vi "EloMec Tester.vi"() -> ()   [LabVIEW 2023]
uses:
  Communication_class/Paths/Convert AI Robot to Robot Command Folder/grSim/grSim Robot Command.ctl
  Communication_class/feedbackData.ctl
  <vilib>/Instr/_visa.llb/VISA Configure Serial Port (Instr).vi
  Communication_class/Communication.lvclass
panel:
  out "Waveform Chart 3":u32(graph)
  out "Waveform Chart 2":u32(graph)
  in  "Modo":T1(ring)
  out "Battery":sgl(graph)
  in  "Feedback ID":u32
  out "Space":bool
  out "kickCharged":bool
  out "hasBall":bool
  out "E":bool
  out "Q":bool
  in  "Keyboard":bool=TRUE
  out "A":bool
  out "D":bool
  out "S":bool
  out "W":bool
  in  "Zero":bool
  out "Waveform Chart":T2(graph)
  out "FeedbackData":T3 {"status" format="%08x"}
  in  "FIRASim?":bool
  in  "IDs":u32[](array[numeric])
  out "Output Array":T4[](array[typedef])=[{"id"=0, "kickspeedx"=0.0, "kickspeedz"=0.0, "veltangent"=0.0, "velnormal"=0.0, "velangular"=0.0, "spinner"=FALSE, "wheelspeed"=FALSE, "wheel1"=0.0, "wheel2"=0.0, "wheel3"=0.0, "wheel4"=0.0, "kickangle"=0.0, "spinner_rpm"=0.0}, {"id"=1, "kickspeedx"=0.0, "kickspeedz"=0.0, "veltangent"=0.0, "velnormal"=0.0, "velangular"=0.0, "spinner"=FALSE, "wheelspeed"=FALSE, "wheel1"=0.0, "wheel2"=0.0, "wheel3"=0.0, "wheel4"=0.0, "kickangle"=0.0, "spinner_rpm"=0.0}, {"id"=2, "kickspeedx"=0.0, "kickspeedz"=0.0, "veltangent"=0.0, "velnormal"=0.0, "velangular"=0.0, "spinner"=FALSE, "wheelspeed"=FALSE, "wheel1"=0.0, "wheel2"=0.0, "wheel3"=0.0, "wheel4"=0.0, "kickangle"=0.0, "spinner_rpm"=0.0}, {"id"=3, "kickspeedx"=0.0, "kickspeedz"=0.0, "veltangent"=0.0, "velnormal"=0.0, "velangular"=0.0, "spinner"=FALSE, "wheelspeed"=FALSE, "wheel1"=0.0, "wheel2"=0.0, "wheel3"=0.0, "wheel4"=0.0, "kickangle"=0.0, "spinner_rpm"=0.0}, {"id"=4, "kickspeedx"=0.0, "kickspeedz"=0.0, "veltangent"=0.0, "velnormal"=0.0, "velangular"=0.0, "spinner"=FALSE, "wheelspeed"=FALSE, "wheel1"=0.0, "wheel2"=0.0, "wheel3"=0.0, "wheel4"=0.0, "kickangle"=0.0, "spinner_rpm"=0.0}, {"id"=5, "kickspeedx"=0.0, "kickspeedz"=0.0, "veltangent"=0.0, "velnormal"=0.0, "velangular"=0.0, "spinner"=FALSE, "wheelspeed"=FALSE, "wheel1"=0.0, "wheel2"=0.0, "wheel3"=0.0, "wheel4"=0.0, "kickangle"=0.0, "spinner_rpm"=0.0}, {"id"=6, "kickspeedx"=0.0, "kickspeedz"=0.0, "veltangent"=0.0, "velnormal"=0.0, "velangular"=0.0, "spinner"=FALSE, "wheelspeed"=FALSE, "wheel1"=0.0, "wheel2"=0.0, "wheel3"=0.0, "wheel4"=0.0, "kickangle"=0.0, "spinner_rpm"=0.0}]
  in  "chip kick":bool
  in  "kickspeedz":sgl=100.0
  in  "drible":bool
  in  "velangular":sgl=5.0
  in  "velnormal":sgl=1.0
  in  "veltangent":sgl=1.0
  in  "kick":bool
  in  "kickspeedx":sgl=100.0
  out "Numeric 2":u32
  out "String":string
  out "return count":u32
  in  "stop":bool
  out "string":string
  out "error out":errorcluster
  in  "termination char\n(0xA = '\\n' = LF)":u8=10 format="%.0x"
  in  "VISA resource name":refnum<visa-resource-name>="COM6"
  in  "Serial Settings":T5={"baud rate"=9600, "data bits"=8, "parity"=enum."None", "stop bits"=10, "flow control"=0} {"flow control" items=["None"=0, "XON/XOFF"=1, "RTS/CTS"=2, "DTR/DSR"=4]; "stop bits" items=["1"=10, "1.5"=15, "2.0"=20]; "data bits" min=5 max=8 step=1; "baud rate" items=["75"=75, "110"=110, "134"=134, "150"=150, "300"=300, "600"=600, "1200"=1200, "1800"=1800, "2400"=2400, "4800"=4800, "7200"=7200, "9600"=9600, "14400"=14400, "19200"=19200, "28800"=28800, "38400"=38400, "56000"=56000, "57600"=57600, "115200"=115200, "128000"=128000, "230400"=230400]}
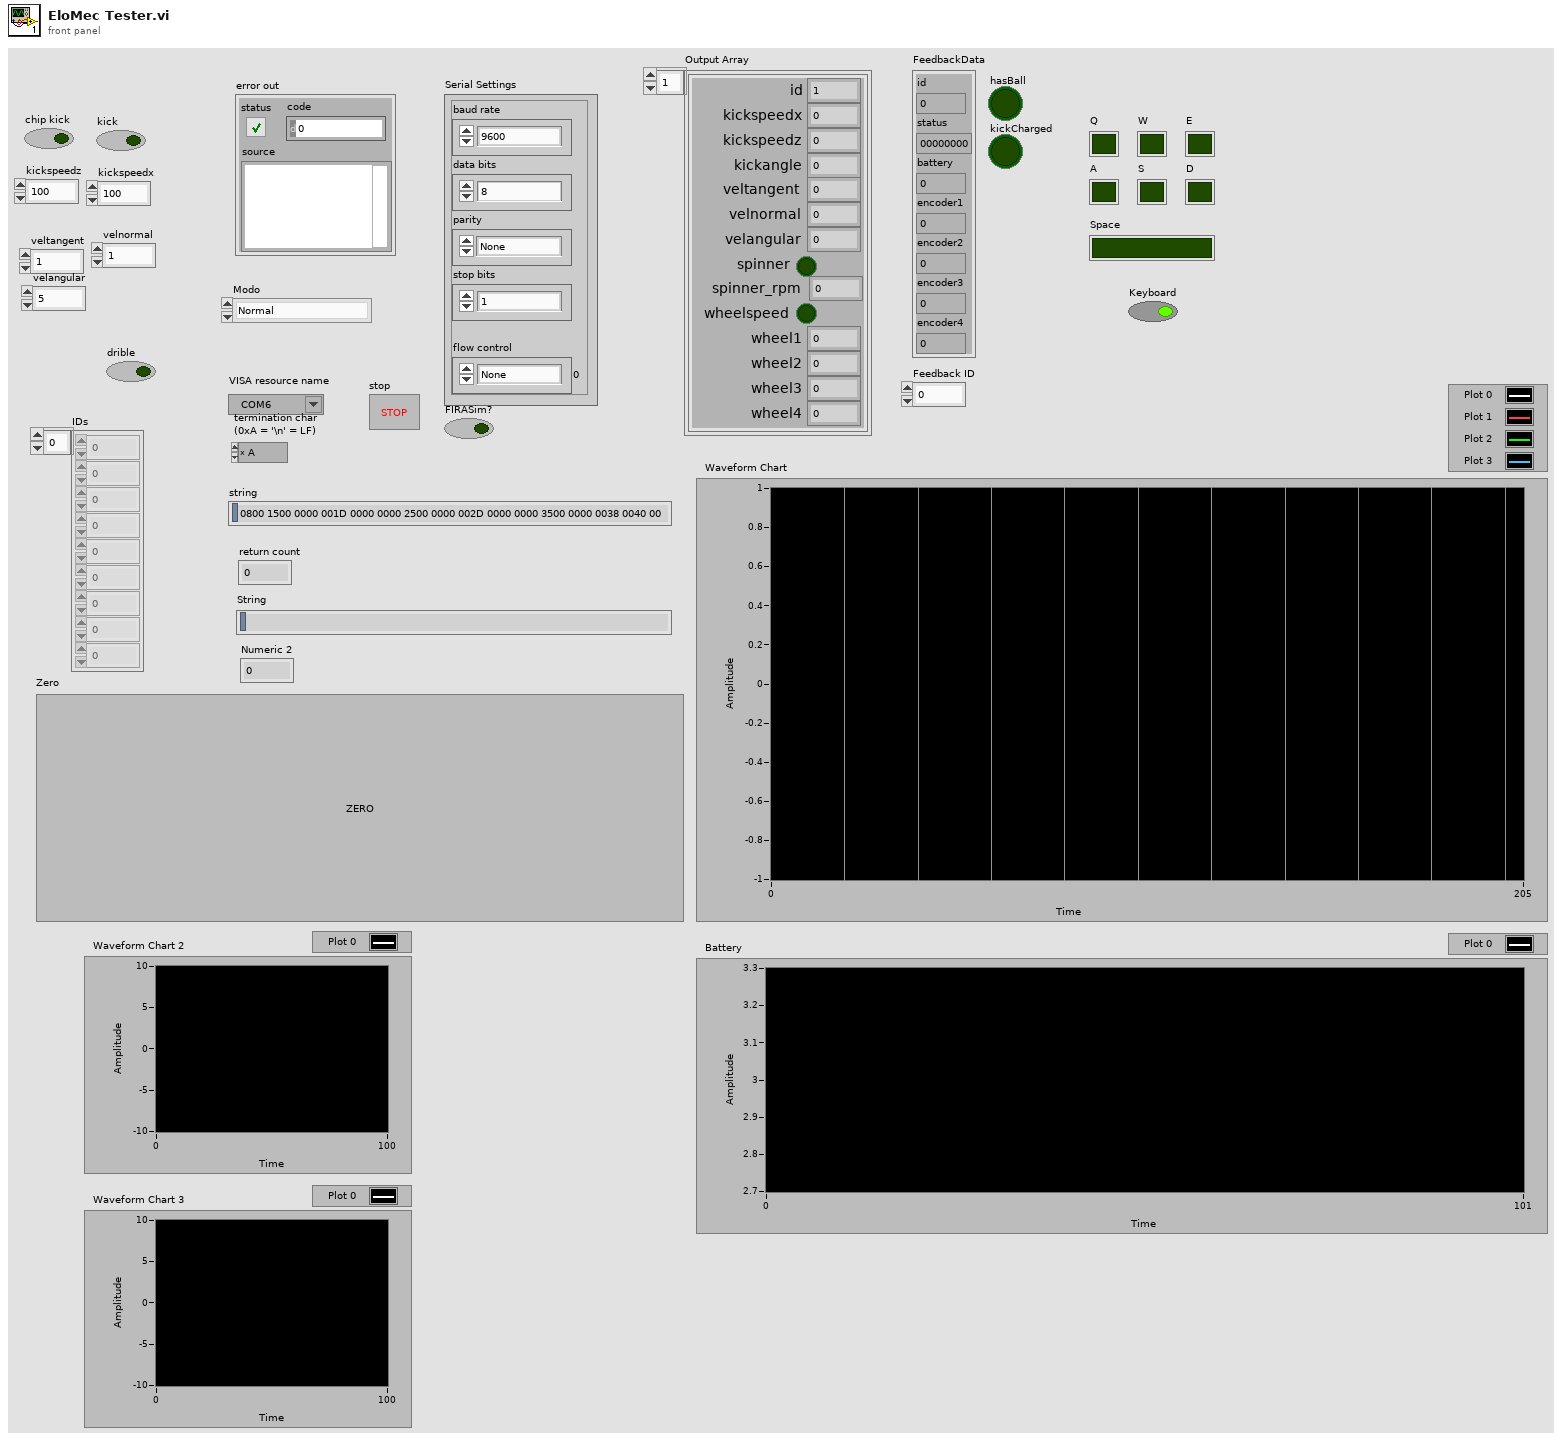
[diagram p1: front panel]
types:
  T1 = enum16{"Normal", "Rampa invertida", "Teste de engrenagem", "Rampa"}
  T2 = cluster{"[0]":sgl, "[1]":sgl, "[2]":sgl, "[3]":sgl, "[4]":sgl, "[5]":sgl, "[6]":sgl, "[7]":sgl, "[8]":sgl}
  T3 = typedef "feedbackData.ctl" = cluster{"id":u32, "status":u32, "battery":sgl, "encoder1":sgl, "encoder2":sgl, "encoder3":sgl, "encoder4":sgl}
  T4 = typedef "grSim Robot Command.ctl" = cluster{"id":u32, "kickspeedx":sgl, "kickspeedz":sgl, "veltangent":sgl, "velnormal":sgl, "velangular":sgl, "spinner":bool, "wheelspeed":bool, "wheel1":sgl, "wheel2":sgl, "wheel3":sgl, "wheel4":sgl, "kickangle":sgl, "spinner_rpm":sgl}
  T5 = cluster{"baud rate":u32, "data bits":u16, "parity":enum16{"None", "Odd", "Even", "Mark", "Space"}, "stop bits":u16, "flow control":u16}
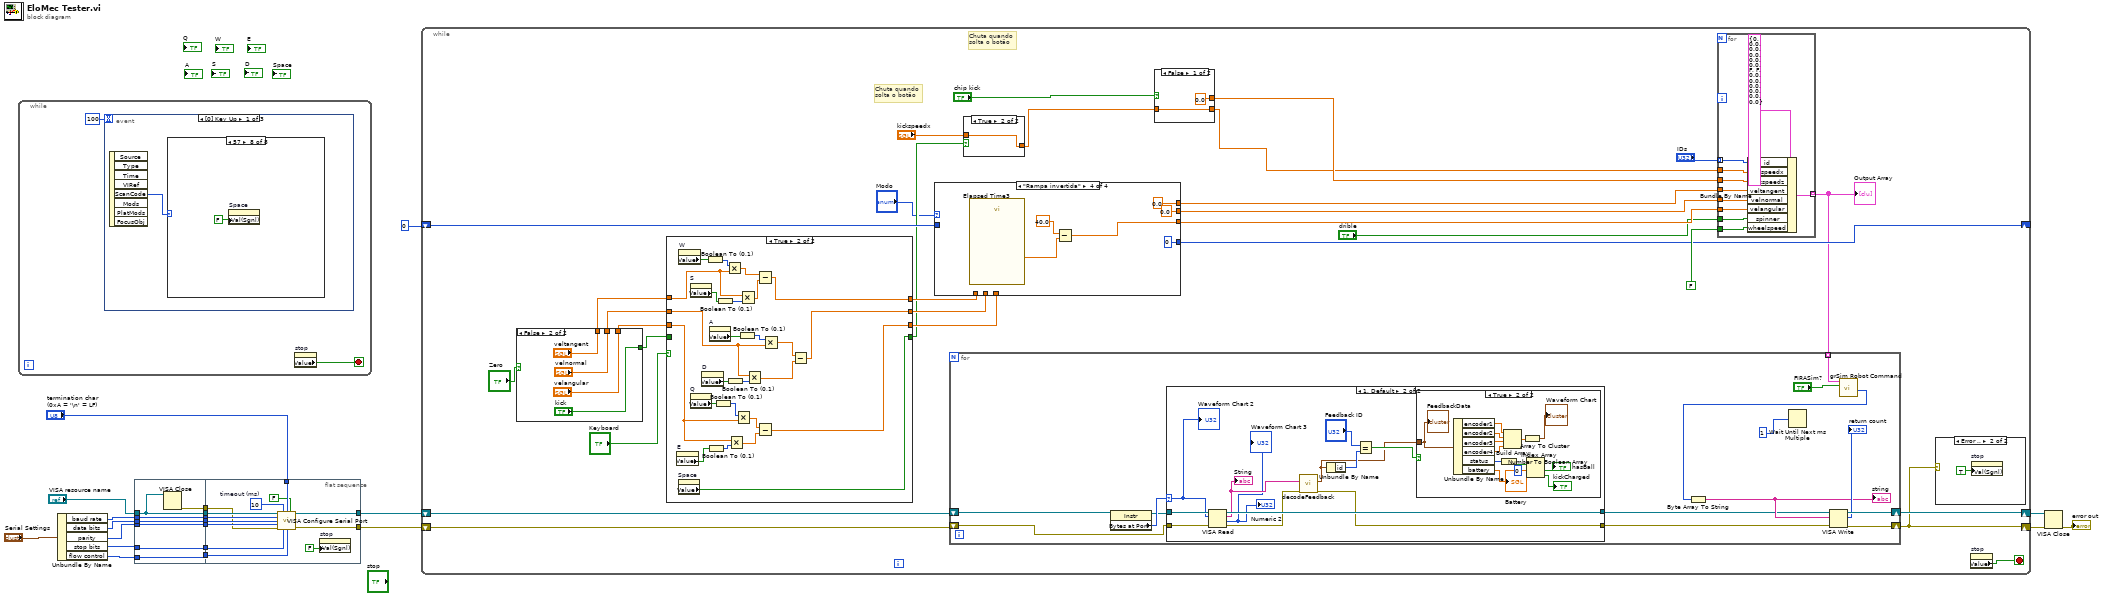
[diagram p0: block diagram]
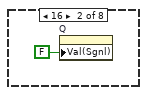
[diagram p3: hidden frame]
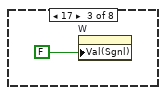
[diagram p4: hidden frame]
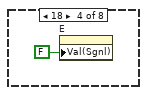
[diagram p5: hidden frame]
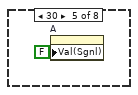
[diagram p6: hidden frame]
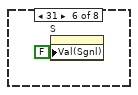
[diagram p7: hidden frame]
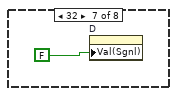
[diagram p8: hidden frame]
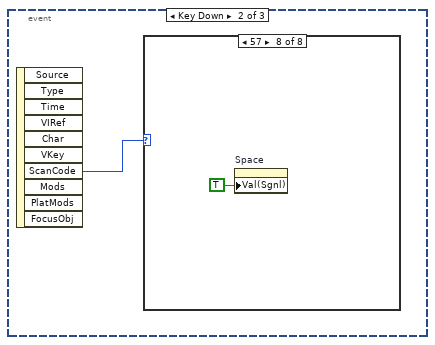
[diagram p9: hidden frame]
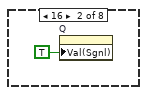
[diagram p11: hidden frame]
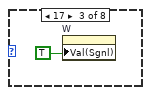
[diagram p12: hidden frame]
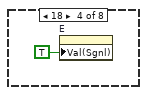
[diagram p13: hidden frame]
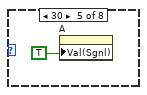
[diagram p14: hidden frame]
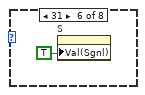
[diagram p15: hidden frame]
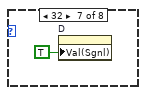
[diagram p16: hidden frame]
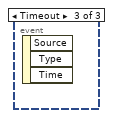
[diagram p17: hidden frame]
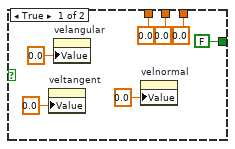
[diagram p20: hidden frame]
diagram:
  n1 = while {
    stop <- w23 stop-if-true
    n2 = event shown="[0] Key Up" {
      selector: _ -> [_ _ _]
      dyn-events: _ -> [_ _ _]
      timeout: 100 -> [_ _ _]
      event Key Up {
        n3 = event-data() -> ("ScanCode"=w24:i16)  [unwired: 1 in, 7 out]
        n4 = case shown="57" w24 {
          frame Default {
          }
          frame 16 {
            n5 = property on="Q" class="Bool (strict)"("Val(Sgnl)"=FALSE ("Value (Signaling)")) -> ()  [unwired: 2 in, 2 out]
          }
          frame 17 {
            n6 = property on="W" class="Bool (strict)"("Val(Sgnl)"=FALSE ("W")) -> ()  [unwired: 2 in, 2 out]
          }
          frame 18 {
            n7 = property on="E" class="Bool (strict)"("Val(Sgnl)"=FALSE ("Value (Signaling)")) -> ()  [unwired: 2 in, 2 out]
          }
          frame 30 {
            n8 = property on="A" class="Bool (strict)"("Val(Sgnl)"=FALSE ("A")) -> ()  [unwired: 2 in, 2 out]
          }
          frame 31 {
            n9 = property on="S" class="Bool (strict)"("Val(Sgnl)"=FALSE ("S")) -> ()  [unwired: 2 in, 2 out]
          }
          frame 32 {
            n10 = property on="D" class="Bool (strict)"("Val(Sgnl)"=FALSE ("D")) -> ()  [unwired: 2 in, 2 out]
          }
          frame 57 {
            n11 = property on="Space" class="Bool (strict)"("Val(Sgnl)"=FALSE ("Value (Signaling)")) -> ()  [unwired: 2 in, 2 out]
          }
        }
      }
      event Key Down {
        n12 = event-data() -> ("ScanCode"=w32:i16)  [unwired: 1 in, 9 out]
        n13 = case shown="57" w32 {
          frame Default {
          }
          frame 16 {
            n14 = property on="Q" class="Bool (strict)"("Val(Sgnl)"=TRUE ("Value (Signaling)")) -> ()  [unwired: 2 in, 2 out]
          }
          frame 17 {
            n15 = property on="W" class="Bool (strict)"("Val(Sgnl)"=TRUE) -> ()  [unwired: 2 in, 2 out]
          }
          frame 18 {
            n16 = property on="E" class="Bool (strict)"("Val(Sgnl)"=TRUE ("Value (Signaling)")) -> ()  [unwired: 2 in, 2 out]
          }
          frame 30 {
            n17 = property on="A" class="Bool (strict)"("Val(Sgnl)"=TRUE) -> ()  [unwired: 2 in, 2 out]
          }
          frame 31 {
            n18 = property on="S" class="Bool (strict)"("Val(Sgnl)"=TRUE) -> ()  [unwired: 2 in, 2 out]
          }
          frame 32 {
            n19 = property on="D" class="Bool (strict)"("Val(Sgnl)"=TRUE) -> ()  [unwired: 2 in, 2 out]
          }
          frame 57 {
            n20 = property on="Space" class="Bool (strict)"("Val(Sgnl)"=TRUE ("Value (Signaling)")) -> ()  [unwired: 2 in, 2 out]
          }
        }
      }
      event Timeout {
        n21 = event-data() -> ()  [unwired: 1 in, 3 out]
      }
    }
    n22 = property on="stop" class="Bool (strict)"() -> ("Value"=w23:bool)  [unwired: 2 in, 2 out]
  }
  n23 = Unbundle By Name("Serial Settings") -> ("baud rate"=w20:u32, "data bits"=w19:u16, "parity"=w18:enum16{"None", "Odd", "Even", "Mark", "Space"}, "stop bits"=w17:u16, "flow control"=w16:u16)
  n24 = flat-sequence {
    tunnel: "VISA resource name" -> [w41]
    tunnel: w16 -> [w42]
    tunnel: w17 -> [w43]
    tunnel: w18 -> [w44]
    tunnel: w19 -> [w45]
    tunnel: w20 -> [w46]
    tunnel: [w46] -> w8
    tunnel: [w45] -> w7
    tunnel: [w44] -> w6
    tunnel: [w43] -> w5
    tunnel: [w42] -> w4
    tunnel: [w41] -> w3
    tunnel: [w40] -> w2
    tunnel: "termination char\n(0xA = '\\n' = LF)" -> [w53]
    tunnel: [w51] -> w13
    tunnel: [w50] -> w11
    tunnel: w8 -> [w59]
    tunnel: w7 -> [w58]
    tunnel: w6 -> [w57]
    tunnel: w5 -> [w56]
    tunnel: w4 -> [w55]
    tunnel: w3 -> [w54]
    tunnel: w2 -> [w48]
    frame #0 {
      n25 = VISA Close(VISA resource name=w41) -> (error out=w40:errorcluster)  [unwired: 1 in]
    }
    frame #1 {
      w49 = u32 10  # timeout (ms)
      n26 = call-poly "VISA Configure Serial Port"("VISA resource name"=w54, "timeout (10sec)"=w49, "termination char\n(0xA = '\\n' = LF)"=w53, "Enable Termination\nChar (T)"=FALSE ("Enable Termination\nChar (T)"), "baud rate (9600)"=w59, "data bits (8)"=w58, "parity (0:none)"=w57, "error in (no error)"=w48, "stop bits (10: 1 bit)"=w56, "flow control (0:none)"=w55) -> ("VISA resource name out"=w51:refnum<visa-resource-name>, "error out"=w50:errorcluster)  [unwired: 4 in]
      n27 = property on="stop" class="Bool (strict)"("Val(Sgnl)"=FALSE ("Value (Signaling)")) -> ()  [unwired: 2 in, 2 out]
    }
  }
  n28 = while {
    shift-right: [w89] -> w12
    shift-left: w13 -> [w64]
    shift-right: [w69] -> w10
    shift-left: w11 -> [w63]
    shift-right: [w82] -> _
    shift-left: 0 -> [w83]
    stop <- w70 stop-if-true
    # "Chuta quando \nsolta o botão"
    # "Chuta quando \nsolta o botão"
    n29 = case shown="False" "Zero" {
      tunnel: [sgl 0.0 ("veltangent") "veltangent"] -> w74
      tunnel: [sgl 0.0 ("velnormal") "velnormal"] -> w75
      tunnel: [sgl 0.0 ("velangular") "velangular"] -> w76
      tunnel: [FALSE ("kick") "kick"] -> w67
      frame True {
        n30 = property on="veltangent" class="DigNum (strict)"("Value"=sgl 0.0 ("veltangent")) -> ()  [unwired: 2 in, 2 out]
        n31 = property on="velangular" class="DigNum (strict)"("Value"=sgl 0.0 ("velangular")) -> ()  [unwired: 2 in, 2 out]
        n32 = property on="velnormal" class="DigNum (strict)"("Value"=sgl 0.0 ("velnormal")) -> ()  [unwired: 2 in, 2 out]
      }
      frame False {
      }
    }
    n33 = case shown="True" "Keyboard" {
      tunnel: w76 -> [w92 w114]
      tunnel: w75 -> [w93 w98]
      tunnel: w74 -> [w94 w107]
      tunnel: [w94 w104] -> w73
      tunnel: [w93 w96] -> w72
      tunnel: [w92 w112] -> w71
      tunnel: w67 -> [w91 _]
      tunnel: [w91 w95] -> w66
      frame False {
      }
      frame True {
        n34 = property on="E" class="Bool (strict)"() -> ("Value"=w118:bool)  [unwired: 2 in, 2 out]
        n35 = property on="Space" class="Bool (strict)"() -> ("Value"=w95:bool)  [unwired: 2 in, 2 out]
        n36 = property on="W" class="Bool (strict)"() -> ("Value"=w111:bool)  [unwired: 2 in, 2 out]
        n37 = property on="S" class="Bool (strict)"() -> ("Value"=w109:bool)  [unwired: 2 in, 2 out]
        n38 = property on="Q" class="Bool (strict)"() -> ("Value"=w119:bool)  [unwired: 2 in, 2 out]
        n39 = property on="D" class="Bool (strict)"() -> ("Value"=w100:bool)  [unwired: 2 in, 2 out]
        n40 = Boolean To (0,1)(Boolean=w111) -> (0, 1=w110:i16)
        n41 = Boolean To (0,1)(Boolean=w118) -> (0, 1=w115:i16)
        n42 = property on="A" class="Bool (strict)"() -> ("Value"=w103:bool)  [unwired: 2 in, 2 out]
        n43 = Boolean To (0,1)(Boolean=w119) -> (0, 1=w117:i16)
        n44 = Boolean To (0,1)(Boolean=w109) -> (0, 1=w108:i16)
        n45 = Multiply(x=w110, y=w107) -> (x*y=w106:sgl)
        n46 = Boolean To (0,1)(Boolean=w100) -> (0, 1=w99:i16)
        n47 = Multiply(x=w114, y=w115) -> (x*y=w113:sgl)
        n48 = Multiply(x=w117, y=w114) -> (x*y=w116:sgl)
        n49 = Boolean To (0,1)(Boolean=w103) -> (0, 1=w102:i16)
        n50 = Multiply(x=w107, y=w108) -> (x*y=w105:sgl)
        n51 = Multiply(x=w98, y=w99) -> (x*y=w97:sgl)
        n52 = Subtract(x=w106, y=w105) -> (x-y=w104:sgl)
        n53 = Subtract(x=w116, y=w113) -> (x-y=w112:sgl)
        n54 = Multiply(x=w102, y=w98) -> (x*y=w101:sgl)
        n55 = Subtract(x=w101, y=w97) -> (x-y=w96:sgl)
      }
    }
    n56 = case shown="\"Rampa invertida\"" "Modo" {
      tunnel: [w189 sgl 0.0 ("veltangent") sgl 0.0 ("veltangent") sgl 0.0 ("veltangent")] -> w87
      tunnel: w73 -> [w189 _ _ _]
      tunnel: [w188 w190 sgl 0.0 ("velnormal") sgl 0.0 ("velnormal")] -> w86
      tunnel: w72 -> [w188 w191 _ _]
      tunnel: w71 -> [w187 _ _ _]
      tunnel: [w187 sgl 0.0 ("velangular") w209 w213] -> w85
      tunnel: w83 -> [_ w196 _ _]
      tunnel: [0 w195 0 0] -> w82
      frame "Normal" {
      }
      frame "Teste de engrenagem" {
        n57 = call "Elapsed Time"() -> ("Time has Elapsed"=w199:bool)  [unwired: 12 in, 7 out]
        n58 = case shown="False" w199 {
          tunnel: w196 -> [w203 w205]
          tunnel: [w203 w204] -> w195
          frame False {
          }
          frame True {
            n59 = Increment(x=w205) -> (x+1=w204:i32)
          }
        }
        n60 = Quotient & Remainder(x=w195, y=2) -> (x-y*floor(x/y)=w193:i32)  [unwired: 1 out]
        n61 = Equal To 0?(x=w193) -> (x = 0?=w192:bool)
        n62 = case shown="True" w192 {
          tunnel: w191 -> [w201 w202]
          tunnel: [w200 w202] -> w190
          frame False {
            n63 = Negate(x=w201) -> (-x=w200:sgl)
          }
          frame True {
          }
        }
      }
      frame "Rampa" {
        n64 = call "Elapsed Time2"() -> ("Elapsed Time (s)"=w209:dbl)  [unwired: 12 in, 7 out]
      }
      frame "Rampa invertida" {
        n65 = call "Elapsed Time3"() -> ("Elapsed Time (s)"=w214:dbl)  [unwired: 12 in, 7 out]
        n66 = Subtract(x=40.0, y=w214) -> (x-y=w213:dbl)
      }
    }
    n67 = case shown="True" w66 {
      tunnel: [sgl 0.0 ("kickspeedx") w217] -> w61
      tunnel: "kickspeedx" -> [_ w217]
      frame False {
      }
      frame True {
      }
    }
    n68 = case shown="False" "chip kick" {
      tunnel: [sgl 0.0 ("kickspeedx") "kickspeedz"] -> w81
      tunnel: w61 -> [w182 w184]
      tunnel: [w182 w184] -> w60
      frame False {
      }
      frame True {
      }
    }
    n69 = for {
      tunnel: FALSE -> [w181]
      tunnel: w60 -> [w180]
      tunnel: w87 -> [w179]
      tunnel: w86 -> [w178]
      tunnel: w85 -> [w177]
      tunnel: "drible" -> [w176]
      tunnel: w81 -> [w175]
      tunnel: [w174] -> w79 mode=indexing
      tunnel: "IDs" -> [w172] mode=indexing
      n70 = Bundle By Name(cluster=T4 {"id"=0, "kickspeedx"=0.0, "kickspeedz"=0.0, "veltangent"=0.0, "velnormal"=0.0, "velangular"=0.0, "spinner"=FALSE, "wheelspeed"=FALSE, "wheel1"=0.0, "wheel2"=0.0, "wheel3"=0.0, "wheel4"=0.0, "kickangle"=0.0, "spinner_rpm"=0.0} ("Robots"), "id"=w172, "kickspeedx"=w180, "kickspeedz"=w175, "veltangent"=w179, "velnormal"=w178, "velangular"=w177, "spinner"=w176, "wheelspeed"=w181) -> (w174:T4)
    }
    "Output Array" <- w79
    n71 = for {
      shift-right: [w142] -> w69
      shift-left: w63 -> [w133]
      shift-right: [w144] -> w89
      shift-left: w64 -> [w134]
      tunnel: w79 -> [w139] mode=indexing
      n72 = property class="Instr"(reference=w134) -> (reference out=w132:refnum<visa-resource-name>, "Bytes at Port"=w137:u32)  [unwired: 1 in, 1 out]
      n73 = case shown="1, Default" w137 {
        selector: w137 -> [_ w148]
        tunnel: w133 -> [w145 w158]
        tunnel: [w145 w154] -> w136
        tunnel: w132 -> [w146 w149]
        tunnel: [w146 w157] -> w135
        frame 0 {
        }
        frame 1, Default {
          n74 = VISA Read(VISA resource name=w149, byte count=w148, error in (no error)=w158) -> (VISA resource name out=w157:refnum<visa-resource-name>, read buffer=w156:string, return count=→"Numeric 2" →"Waveform Chart 3":u32, error out=w155:errorcluster)
          "String" <- w156
          n75 = call "decodeFeedback.vi"("error in (no error)"=w155, "String"=w156) -> ("error out"=w154:errorcluster, "FeedbackData"=w150:T3)  [unwired: 7 in, 1 out]
          n76 = Unbundle By Name(w150) -> ("id"=w152:u32)
          n77 = Equal?(x="Feedback ID", y=w152) -> (x = y?=w151:bool)
          n78 = case shown="True" w151 {
            tunnel: w150 -> [_ w161]
            frame False {
            }
            frame True {
              n79 = Unbundle By Name(w161) -> ("encoder1"=w160:sgl, "encoder2"=w171:sgl, "encoder3"=w170:sgl, "encoder4"=w169:sgl, "status"=w166:u32, "battery"=→"Battery":sgl)
              n80 = Number To Boolean Array(number=w166) -> (Boolean array=w165:bool[])
              n81 = Build Array(w160, w171, w170, w169) -> (w168:sgl[])
              n82 = Array To Cluster(array=w168) -> (cluster=→"Waveform Chart":T2)
              n83 = Index Array(array=w165, index #1=0 ("index")) -> (element #1=→"hasBall":bool, element #2=→"kickCharged":bool)  [unwired: 1 in]
              "FeedbackData" <- w161
            }
          }
          "Waveform Chart 2" <- w148
        }
      }
      n84 = Wait Until Next ms Multiple(millisecond multiple=u32 1 ("milliseconds to wait")) -> ()  [unwired: 1 out]
      n85 = call "grSim Robot Command.vi"("FIRASim?"="FIRASim?", "Robots"=w139) -> ("Array"=w140:u8[])  [unwired: 9 in]
      n86 = Byte Array To String(unsigned byte array=w140) -> (string=w141:string)
      "string" <- w141
      n87 = VISA Write(VISA resource name=w135, write buffer=w141, error in (no error)=w136) -> (VISA resource name out=w144:refnum<visa-resource-name>, return count=→"return count":u32, error out=w142:errorcluster)
    }
    n88 = case shown="Error .." w69 {
      frame No Error {
      }
      frame Error {
        n89 = property on="stop" class="Bool (strict)"("Val(Sgnl)"=TRUE ("Value (Signaling)")) -> ()  [unwired: 2 in, 2 out]
      }
    }
    n90 = property on="stop" class="Bool (strict)"() -> ("Value"=w70:bool)  [unwired: 2 in, 2 out]
  }
  n91 = VISA Close(VISA resource name=w12, error in (no error)=w10) -> (error out=→"error out":errorcluster)
